vi "Read Variant Data.vi"(8 "error in (no error)":errorcluster, 11 "Base in":refnum<class "Base.lvclass">) -> (0 "error out":errorcluster, 2 "data":variant, 3 "Base out":refnum<class "Base.lvclass">)   [LabVIEW 2020, in "PV Access.lvlib" / "PV Data.lvlib" / "Base.lvclass"]
uses:
  Base.lvclass
  Base.lvclass/Base.ctl
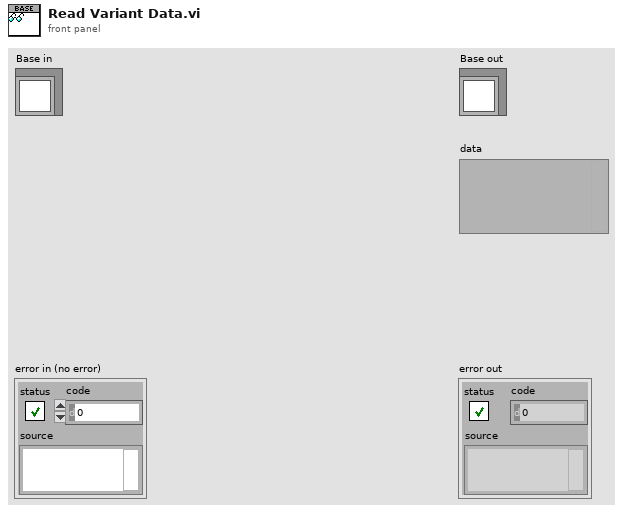
[diagram p1: front panel]
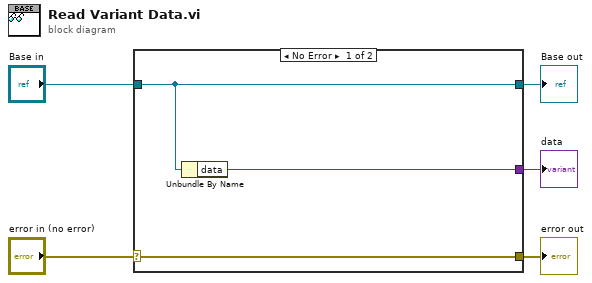
[diagram p0: block diagram]
diagram:
  n1 = case shown="No Error" "error in (no error)" {
    selector: "error in (no error)" -> [w8 w9]
    tunnel: [w8 w9] -> w4
    tunnel: [w7 w10] -> w2
    tunnel: "Base in" -> [w7 w10]
    tunnel: [w6 _] -> w1
    frame No Error {
      n2 = Unbundle By Name(w7) -> ("data"=w6:variant)
    }
    frame Error {
    }
  }
  "error out" <- w4
  "Base out" <- w2
  "data" <- w1
